vi "p2.vi"() -> ()   [LabVIEW 2025, in "d11.lvlib"]
uses:
  d11.lvlib
  lv2025-aoc/AOC/Graph/Graph.lvclass
  lv2025-aoc/AOC/Topological Sort/Topological Sort.lvclass
  lv2025-aoc/AOC/AOC.lvlib
panel:
  in  "Example":string="svr: aaa bbb\naaa: fft\nfft: ccc\nbbb: tty\ntty: ccc\nccc: ddd eee\nddd: hub\nhub: fff\neee: dac\ndac: fff\nfff: ggg hhh\nggg: out\nhhh: out"
  in  "Example 2":bool
  out "Answer":u64
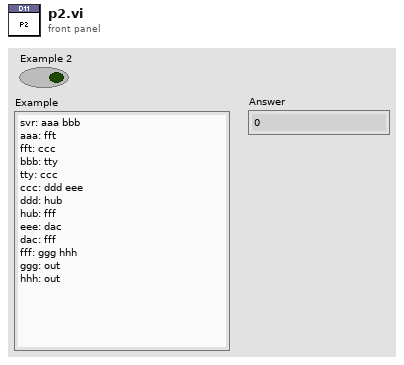
[diagram p1: front panel]
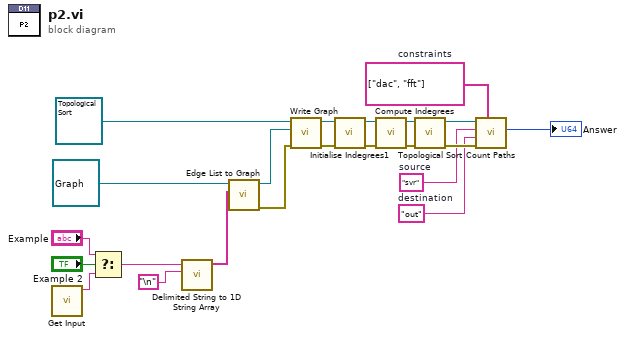
[diagram p0: block diagram]
diagram:
  w14 = string[] ["dac", "fft"]  # constraints
  w1 = "out"  # destination
  w2 = "svr"  # source
  n1 = call "Get Input.vi"() -> ("Input"=w22:string)  [unwired: 11 in]
  n2 = Select(t="Example", s="Example 2", f=w22) -> (s? t:f=w19:string)
  n3 = call <vilib>:"Delimited String to 1D String Array.vi"("delimiter"="\n", "delimited string"=w19) -> ("string array"=w12:string[])  [unwired: 9 in]
  n4 = call-dynamic "Edge List to Graph.vi"("Edge List (src: dst0 dst1..dtsn-1)"=w12, "Graph in"=refnum<class "Graph.lvclass"> refnum) -> ("error out"=w7:errorcluster, "Graph out"=w10:refnum<class "Graph.lvclass">)  [unwired: 8 in]
  n5 = call-dynamic "Write Graph.vi"("error in (no error)"=w7, "Graph"=w10, "Topological Sort in"=refnum<class "Topological Sort.lvclass"> refnum) -> ("error out"=w8:errorcluster, "Topological Sort out"=w9:refnum<class "Topological Sort.lvclass">)  [unwired: 7 in]
  n6 = call "Initialise Indegrees1.vi"("error in (no error)"=w8, "Topological Sort in"=w9) -> ("error out"=w6:errorcluster, "Topological Sort out"=w15:refnum<class "Topological Sort.lvclass">)  [unwired: 8 in]
  n7 = call "Compute Indegrees.vi"("error in (no error)"=w6, "Topological Sort in"=w15) -> ("error out"=w5:errorcluster, "Topological Sort out"=w17:refnum<class "Topological Sort.lvclass">)  [unwired: 8 in]
  n8 = call "Topological Sort.vi"("error in (no error)"=w5, "Topological Sort in"=w17) -> ("error out"=w4:errorcluster, "Topological Sort out"=w16:refnum<class "Topological Sort.lvclass">)  [unwired: 8 in]
  n9 = call "Count Paths.vi"("constraints"=w14, "error in (no error)"=w4, "destination"=w1, "source"=w2, "Topological Sort in"=w16) -> ("Number of Paths"=→"Answer":u64)  [unwired: 4 in, 2 out]
